vi "computeTheta.vi"(3 "thetaT":dbl, 4 "M":dbl, 5 "L":dbl) -> (1 "ThetaOut":dbl[](array[numeric]))   [LabVIEW 2018]
panel:
  out "Kr":dbl[](array[numeric])
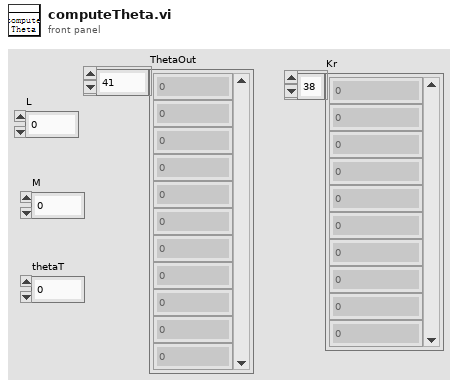
[diagram p1: front panel]
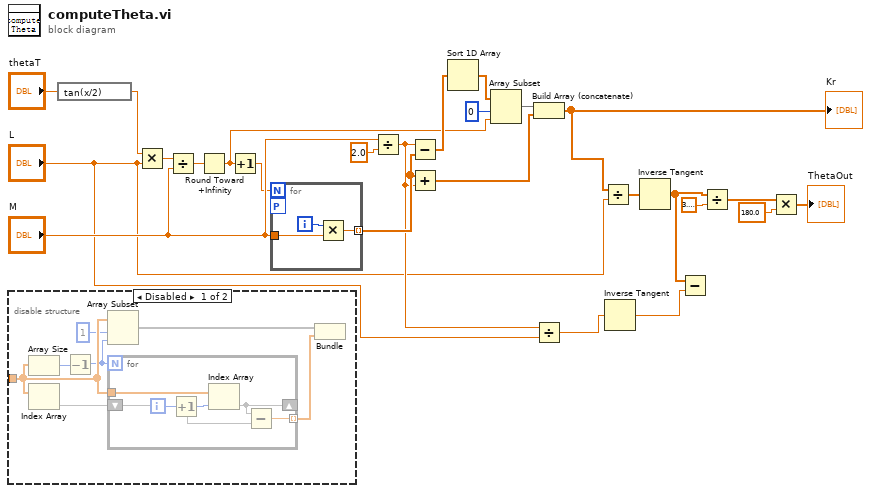
[diagram p0: block diagram]
diagram:
  n1 = disable-structure shown="Disabled" {
    disable-tunnel: _ -> [w30 _]
    frame Disabled {
      n2 = Array Size(array=w30) -> (size(s)=w31:i32)
      n3 = Index Array(array=w30) -> (element=w32)  [unwired: 1 in]
      n4 = Decrement(x=w31) -> (x-1=w28:i32)
      n5 = Array Subset(array=w30, index=1, length=w28) -> (w27:void[])
      n6 = for {
        N: w28 -> [_]
        tunnel: w30 -> [w38]
        tunnel: [w33] -> w26 mode=indexing
        shift-right: [w35] -> _
        shift-left: w32 -> [w34]
        i -> [w37]
        n7 = Increment(x=w37) -> (x+1=w36:i32)
        n8 = Index Array(array=w38, index=w36) -> (element=w35)
        n9 = Subtract(x=w35, y=w34) -> (x-y=w33:dbl)
      }
      n10 = Bundle(w27, w26) -> ()  [unwired: 1 in, 1 out]
    }
    frame Enabled {
    }
  }
  n11 = expression code="tan(x/2)"("thetaT") -> (w23:dbl)
  n12 = Multiply(x=w23, y="L") -> (x*y=w22:dbl)
  n13 = Divide(x=w22, y="M") -> (x/y=w21:dbl)
  n14 = Round Toward +Infinity(x=w21) -> (ceil(x): smallest int >= x=w8:dbl)
  n15 = Increment(x=w8) -> (x+1=w7:dbl)
  n16 = for "For循环" {
    N: w7 -> [_]
    tunnel: "M" -> [w41]
    tunnel: [w40] -> w10 mode=indexing
    workers-P: _ -> [_]
    i -> [w39]
    n17 = Multiply(x=w39, y=w41) -> (x*y=w40:dbl)
  }
  n18 = Divide(x="M", y=2.0) -> (x/y=w5:dbl)
  n19 = Subtract(x=w5, y=w10) -> (x-y=w20:dbl[])
  n20 = Add(x=w10, y=w5) -> (x+y=w12:dbl[])
  n21 = Sort 1D Array(array=w20) -> (sorted array=w14:dbl[])
  n22 = Array Subset(array=w14, index=0, length=w8) -> (w9:dbl[])
  n23 = Build Array (concatenate)(w9, w12) -> (w6:dbl[])
  "Kr" <- w6
  n24 = Divide(x=w5, y="L") -> (x/y=w3:dbl)
  n25 = Divide(x=w6, y="L") -> (x/y=w16:dbl[])
  n26 = Inverse Tangent(1:w3) -> (0:w2:dbl)
  n27 = Inverse Tangent(1:w16) -> (0:w1:dbl[])
  n28 = Subtract(x=w1, y=w2) -> ()  [unwired: 1 out]
  n29 = Divide(x=w1, y=3.141592653589793) -> (x/y=w18:dbl[])
  n30 = Multiply(x=w18, y=180.0) -> (x*y=→"ThetaOut":dbl[])
